vi "Synchronize_Prog_Arg.vi"(5 "Execution Row":T1 {"Carrier_2 Q (l/min)" format="%#.2f"; "Row Duration (mins)" format="%#.1f"; "Row No" min=0; "Trace Gas Concentration (%)" min=0.0 format="%#_4f"; "Carrier_1 Q (l/min)" format="%#.2f"; "Tunnel Speed" format="%#.2f"; "Start X" format="%#.2f"; "Start Y" format="%#.2f"; "Start Z" format="%#.2f"; "End X" format="%#.2f"; "End Y" format="%#.2f"; "End Z" format="%#.2f"; "Averaging time (min)" min=0.0 format="%#.2f"}) -> (0 "Jump to fall back row":bool, 1 "Raise alarm after (mins)":i32, 2 "Error Comments":string, 3 "Machine names":string[](array[string]), 4 "Sync No":i32)   [LabVIEW 2014]
uses:
  Traverse_cluster.ctl
  Spacing.ctl
  Controls/Multi_run_mode.ctl
  Globals/Preference_global.vi
panel:
  # "X           Y            Z"
  # "Start"
  # "End"
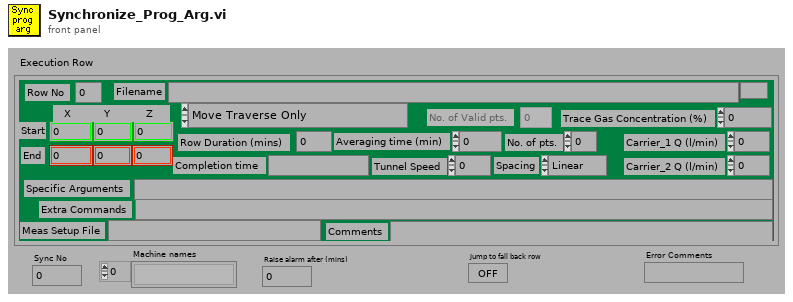
[diagram p1: front panel]
types:
  T1 = typedef "Traverse_cluster.ctl" = cluster{"Start X":sgl, "Start Y":sgl, "Start Z":sgl, "End X":sgl, "End Y":sgl, "End Z":sgl, "No. of pts.":i32, "Spacing":T2, "Filename":path, "Tunnel Speed":dbl, "Averaging time (min)":dbl, "Extra Commands":string, "Carrier_1 Q (l/min)":dbl, "Carrier_2 Q (l/min)":dbl, "Trace Gas Concentration (%)":dbl, "Specific Arguments":string, "Comments":string, "Row No":i32, "Row Type Selector":T3, "Completion time":string, "Row Duration (mins)":dbl, "No. of Valid pts.":i32, "Meas Setup File":string}
  T2 = typedef "Spacing.ctl" = enum16{"Linear", "Log", "Gauss", "Specified", "N/A"}
  T3 = typedef "Multi_run_mode.ctl" = enum16{"Move Traverse Only", "Set Tunnel Speed Only", "Set Source Only", "Set Measurement Conditions", "Single Measurement", "Vertical Profile", "Lateral Profile", "Longitudinal Profile", "Explore Volume", "Multi-Axis Profile", "Auto Calibrate", "Meas Fast FID Bkgnd", "Check Beam Power", "Scanning Valve Measurement", "Run VI Named:", "Set ADAM Ch", "Wait (minutes)", "Send Message", "Synchronize With:", "Fall Back to this Row", "Turn Off Row Repeating", "Blank Row", "Traverse 3D Volume"}
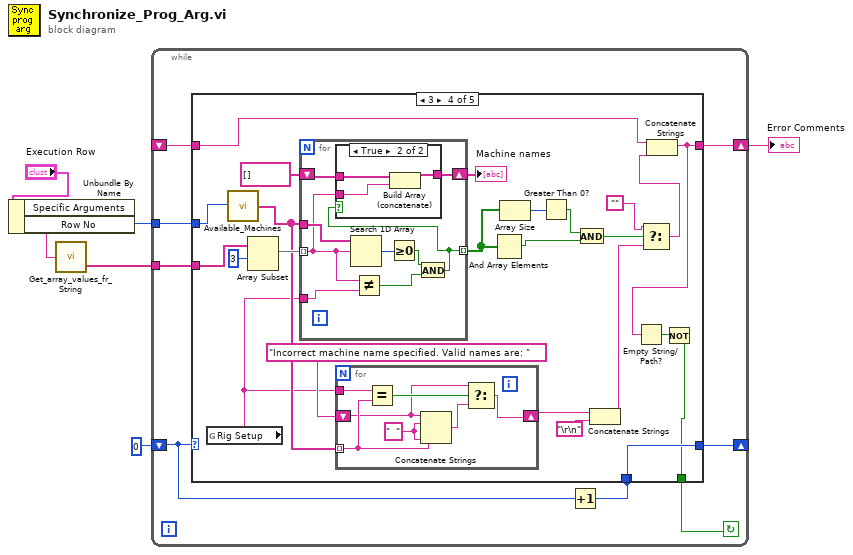
[diagram p0: block diagram]
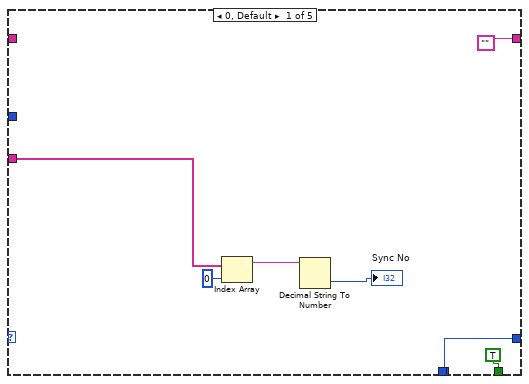
[diagram p2: hidden frame]
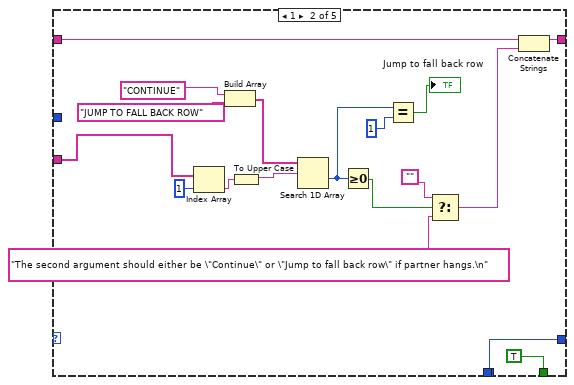
[diagram p3: hidden frame]
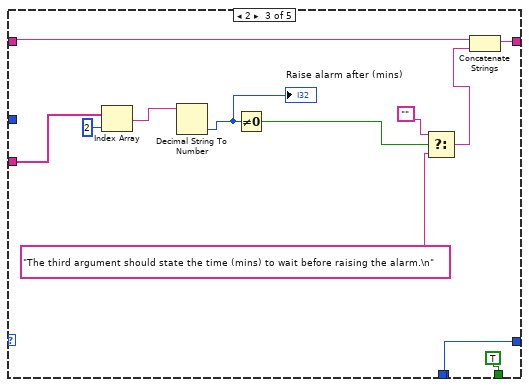
[diagram p4: hidden frame]
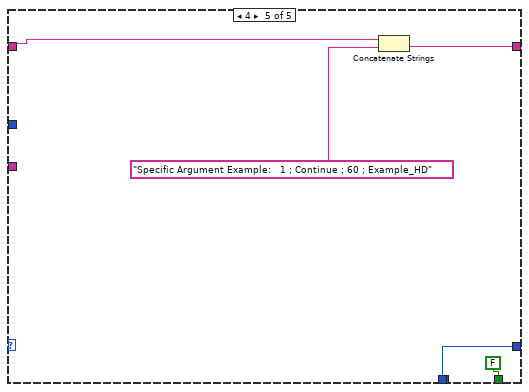
[diagram p6: hidden frame]
diagram:
  n1 = Unbundle By Name("Execution Row") -> ("Specific Arguments"=w6:string, "Row No"=w1:i32)
  n2 = call "Get_array_values_fr_String.vi"("String Value"=w6) -> ("String array"=w3:string[])  [unwired: 1 out]
  n3 = while {
    tunnel: w1 -> [w7]
    shift-left: _ -> [w9]
    shift-right: [w10] -> w2
    tunnel: w3 -> [w14]
    shift-left: 0 -> [w13]
    shift-right: [w12] -> _
    stop <- w11 continue-if-true
    n4 = Increment(x=w13) -> (x+1=w8:i32)
    n5 = case shown="3" w13 {
      tunnel: w14 -> [w18 w27 w40 w61 _]
      tunnel: w8 -> [w17 w26 w45 w64 _]
      tunnel: [w17 w26 w45 w64 w96] -> w12
      tunnel: [TRUE TRUE TRUE w55 FALSE] -> w11
      tunnel: ["" w22 w42 w57 w99] -> w10
      tunnel: w9 -> [_ w24 w43 w62 w100]
      tunnel: w8 -> [_ _ _ _ w96]
      tunnel: w7 -> [_ _ _ w53 _]
      frame 0, Default {
        n6 = Index Array(array=w18, index=0 ("Index")) -> (element=w20:string)
        n7 = Decimal String To Number(string=w20) -> (number=→"Sync No":i32)  [unwired: 3 out]
      }
      frame 1 {
        n8 = Index Array(array=w27, index=1 ("Index")) -> (element=w35:string)
        n9 = Build Array("CONTINUE", "JUMP TO FALL BACK ROW") -> (w33:string[])
        n10 = To Upper Case(1:w35) -> (0:w34:string)
        n11 = Search 1D Array(1D array=w33, element=w34) -> (index of element=w30:i32)  [unwired: 1 out]
        n12 = Greater Or Equal To 0?(x=w30) -> (x >= 0?=w31:bool)
        n13 = Equal?(x=w30, y=1) -> (x = y?=→"Jump to fall back row":bool)
        n14 = Select(t="", s=w31, f="The second argument should either be \"Continue\" or \"Jump to fall back row\" if partner hangs.\n" ("Format String")) -> (s? t:f=w23:string)
        n15 = Concatenate Strings(w24, w23) -> (w22:string)
      }
      frame 2 {
        n16 = Index Array(array=w40, index=2 ("Index")) -> (element=w48:string)
        n17 = Decimal String To Number(string=w48) -> (number=w47:i32)  [unwired: 3 out]
        "Raise alarm after (mins)" <- w47
        n18 = Not Equal To 0?(x=w47) -> (x != 0?=w46:bool)
        n19 = Select(t="", s=w46, f="The third argument should state the time (mins) to wait before raising the alarm.\n" ("Format String")) -> (s? t:f=w41:string)
        n20 = Concatenate Strings(w43, w41) -> (w42:string)
      }
      frame 3 {
        n21 = global read "Preference_global.vi" "Rig Setup"() -> (w52:string)
        n22 = call "Available_Machines.vi"("Row Number"=w53) -> ("Machine Names"=w54:string[])
        n23 = Array Subset(array=w61, index=3 ("Array Index")) -> (w74:string[])  [unwired: 1 in]
        n24 = for {
          tunnel: w54 -> [w91]
          tunnel: w74 -> [w87] mode=indexing
          tunnel: [w83] -> w73 mode=indexing
          shift-right: [w88] -> w66
          shift-left: string[] [] -> [w89]
          tunnel: w52 -> [w86]
          n25 = Search 1D Array(1D array=w91, element=w87) -> (index of element=w90:i32)  [unwired: 1 out]
          n26 = Not Equal?(x=w87, y=w86) -> (x != y?=w84:bool)
          n27 = Greater Or Equal To 0?(x=w90) -> (x >= 0?=w85:bool)
          n28 = And(x=w85, y=w84) -> (x .and. y?=w83:bool)
          n29 = case shown="True" w83 {
            tunnel: w89 -> [w92 w95]
            tunnel: [w92 w94] -> w88
            tunnel: w87 -> [_ w93]
            frame False {
            }
            frame True {
              n30 = Build Array (concatenate)(w95, w93) -> (w94:string[])
            }
          }
        }
        "Machine names" <- w66
        n31 = for {
          shift-right: [w76] -> w60
          shift-left: "Incorrect machine name specified. Valid names are: " -> [w78]
          tunnel: w54 -> [w80] mode=indexing
          tunnel: w52 -> [w81]
          w82 = "  " ("Substring")
          n32 = Equal?(x=w81, y=w80) -> (x = y?=w79:bool)
          n33 = Concatenate Strings(w78, w82, w80, w82) -> (w77:string)
          n34 = Select(t=w78, s=w79, f=w77) -> (s? t:f=w76:string)
        }
        n35 = And Array Elements(Boolean array=w73) -> (logical AND=w70:bool)
        n36 = Array Size(array=w73) -> (size(s)=w72:i32)
        n37 = Greater Than 0?(x=w72) -> (x > 0?=w71:bool)
        n38 = And(x=w71, y=w70) -> (x .and. y?=w69:bool)
        n39 = Concatenate Strings(w60, "\r\n") -> (w59:string)
        n40 = Select(t="", s=w69, f=w59) -> (s? t:f=w63:string)
        n41 = Concatenate Strings(w62, w63) -> (w57:string)
        n42 = Empty String/Path?(string/path=w57) -> (empty?=w56:bool)
        n43 = Not(x=w56) -> (.not. x?=w55:bool)
      }
      frame 4 {
        n44 = Concatenate Strings(w100, "Specific Argument Example:   1 ; Continue ; 60 ; Example_HD") -> (w99:string)
      }
    }
  }
  "Error Comments" <- w2
